vi "CheckTestSelection.vi"(3 "错误输入":errorcluster, 4 "产品型号":refnum<vi>, 5 "测试结果":refnum<vi>[](array[refnum]), 6 "测试选择":refnum<vi>[](array[refnum])) -> (0 "错误输出":errorcluster, 1 "TestPara":cluster{"TestStep":string[], "Enable":bool[]}[](array[cluster]), 2 "ExcelNames":string[](array[string]))   [LabVIEW 2013]
uses:
  <vilib>/Utility/NIReport.llb/NI_report.lvclass
  <vilib>/Utility/NIReport.llb/Excel/NI_Excel.lvclass
panel:
  out "进度条":u8(slide) scale=0.0..100.0
  out "字符串":string="正在检查测试用例配置文件"
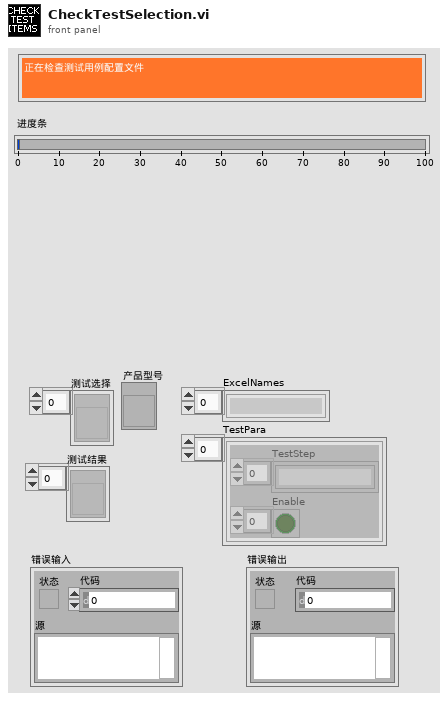
[diagram p1: front panel]
types:
  T1 = enum8{"Enabled", "Disabled", "Disabled and Grayed Out"}
  T2 = enum32{"invalid app kind", "Development System", "Run Time System", "Student Edition", "Embedded LabVIEW", "Evaluation", "Custom"}
  T3 = enum16{"maximized", "minimized", "normal", "no change"}
  T4 = enum16{"Standard Report", "HTML", "Word", "Excel"}
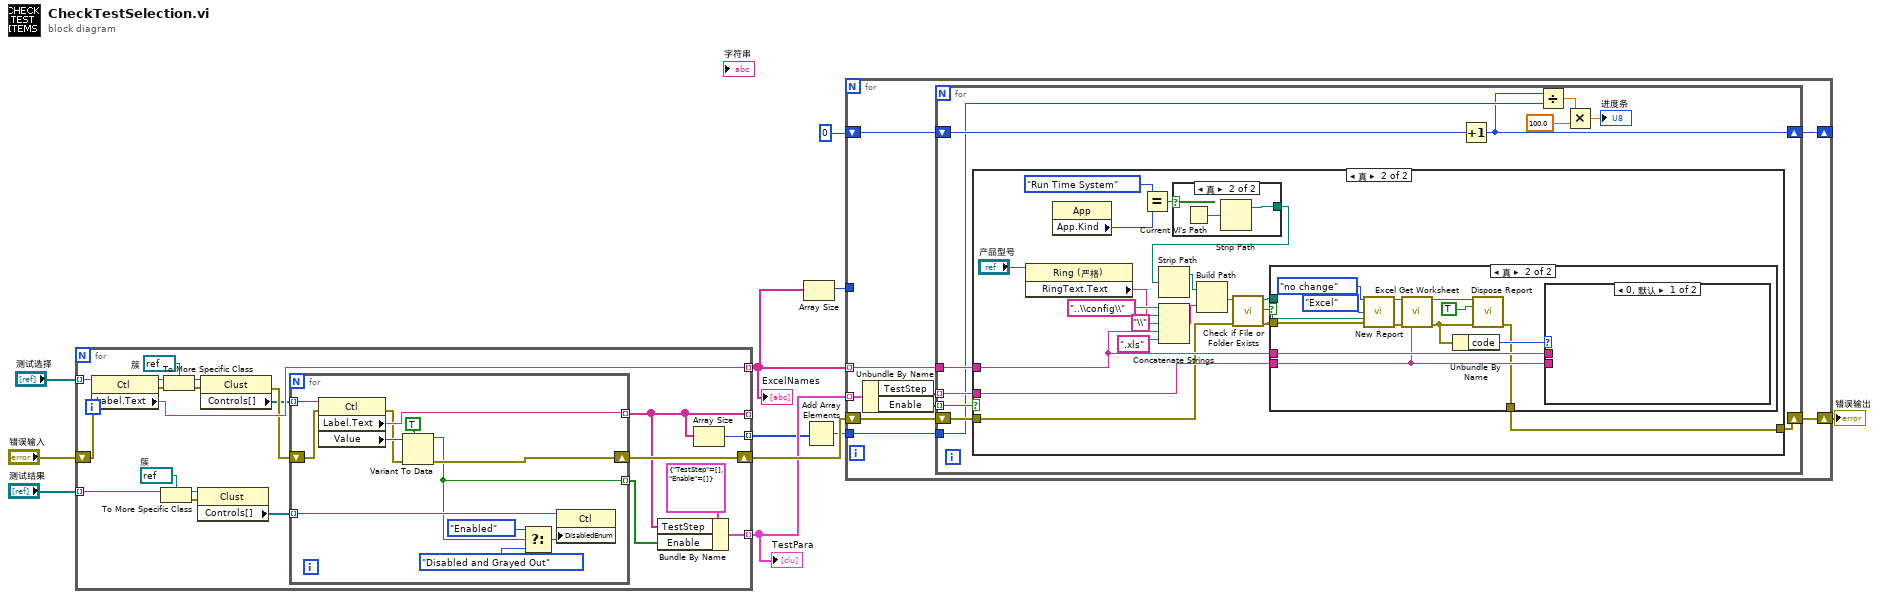
[diagram p0: block diagram]
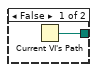
[diagram p3: hidden frame]
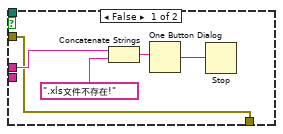
[diagram p4: hidden frame]
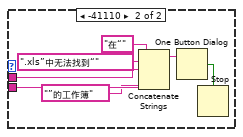
[diagram p5: hidden frame]
diagram:
  n1 = for {
    tunnel: "测试选择" -> [w32] mode=indexing
    tunnel: [w28] -> w5 mode=indexing
    tunnel: [w13] -> _ mode=indexing
    shift-right: [w23] -> w10
    shift-left: "错误输入" -> [w24]
    tunnel: "测试结果" -> [w19] mode=indexing
    tunnel: [w14] -> w6 mode=indexing
    tunnel: [w12] -> w2 mode=indexing
    w20 = refnum<vi> refnum  # 簇
    w30 = refnum<vi> refnum  # 簇
    n2 = property class="Ctl"(reference=w32, error in=w24) -> (reference out=w31:refnum<vi>, error out=w27:errorcluster, "Label.Text"=w28:string)
    n3 = To More Specific Class(target class=w20, reference=w19) -> (specific class reference=w21:refnum<vi>, error out=w22:errorcluster)  [unwired: 1 in]
    n4 = To More Specific Class(target class=w30, reference=w31, error in=w27) -> (specific class reference=w29:refnum<vi>, error out=w26:errorcluster)
    n5 = property class="Clust"(reference=w21, error in=w22) -> ("Controls[]"=w17:refnum<vi>[])  [unwired: 2 out]
    n6 = property class="Clust"(reference=w29, error in=w26) -> (error out=w25:errorcluster, "Controls[]"=w18:refnum<vi>[])  [unwired: 1 out]
    n7 = for {
      tunnel: w18 -> [w44] mode=indexing
      tunnel: [w41] -> w13 mode=indexing
      shift-right: [w38] -> w23
      shift-left: w25 -> [w40]
      tunnel: w17 -> [w37] mode=indexing
      tunnel: [w34] -> w16 mode=indexing
      n8 = property class="Ctl"(reference=w44, error in=w40) -> (error out=w39:errorcluster, "Label.Text"=w41:string, "Value"=w42:variant)  [unwired: 1 out]
      n9 = Variant To Data(error in=w39, type=TRUE, Variant=w42) -> (data=w34:bool, error out=w38:errorcluster)
      n10 = Select(t=T1."Enabled" ("禁用"), s=w34, f=T1."Disabled and Grayed Out" ("禁用")) -> (s? t:f=w33:T1)
      n11 = property class="Ctl"(reference=w37, "DisabledEnum"=w33) -> ()  [unwired: 1 in, 2 out]
    }
    n12 = Bundle By Name(cluster=cluster{"TestStep":string[], "Enable":bool[]} {"TestStep"=[], "Enable"=[]} ("簇"), "TestStep"=w13, "Enable"=w16) -> (w14:cluster{"TestStep":string[], "Enable":bool[]})
    n13 = Array Size(array=w13) -> (size(s)=w12:i32)
  }
  "ExcelNames" <- w5
  "TestPara" <- w6
  n14 = Array Size(array=w5) -> (size(s)=w4:i32)
  n15 = Add Array Elements(numeric array=w2) -> (sum=w1:i32)
  n16 = for {
    tunnel: w5 -> [w53] mode=indexing
    shift-right: [w51] -> w9
    shift-left: w10 -> [w52]
    tunnel: w6 -> [w50] mode=indexing
    tunnel: w4 -> [_]
    shift-right: [w46] -> _
    shift-left: 0 -> [w47]
    tunnel: w1 -> [w45]
    n17 = Unbundle By Name(w50) -> ("TestStep"=w49:string[], "Enable"=w48:bool[])
    n18 = for {
      tunnel: w53 -> [w64]
      shift-right: [w62] -> w51
      shift-left: w52 -> [w63]
      tunnel: w49 -> [w61] mode=indexing
      tunnel: w48 -> [w60] mode=indexing
      shift-right: [w54] -> w46
      shift-left: w47 -> [w59]
      tunnel: w45 -> [w55]
      n19 = case shown="真" w60 {
        tunnel: w64 -> [_ w76]
        tunnel: w61 -> [_ w75]
        tunnel: w63 -> [w65 w74]
        tunnel: [w65 w73] -> w62
        frame False {
        }
        frame True {
          n20 = property class="Ring (严格)"(reference="产品型号") -> ("RingText.Text"=w68:string)  [unwired: 1 in, 2 out]
          n21 = property class="App"() -> ("App.Kind"=w71:T2)  [unwired: 2 in, 2 out]
          n22 = Equal?(x=T2."Run Time System" ("y"), y=w71) -> (x = y?=w70:bool)
          n23 = Concatenate Strings("..\\config\\" ("连接的字符串"), w68, "\\" ("字符串"), w76, ".xls" ("连接的字符串")) -> (w79:string)
          n24 = case shown="真" w70 {
            tunnel: [w85 w87] -> w69
            frame False {
              n25 = Current VI's Path() -> (path=w85:path)
            }
            frame True {
              n26 = Current VI's Path() -> (path=w86:path)
              n27 = Strip Path(path=w86) -> (stripped path=w87:path)  [unwired: 1 out]
            }
          }
          n28 = Strip Path(path=w69) -> (stripped path=w81:path)  [unwired: 1 out]
          n29 = Build Path(base path=w81, name or relative path=w79) -> (appended path=w78:path)
          n30 = call <vilib>:"Check if File or Folder Exists.vi"("error in (no error)"=w74, "path"=w78) -> ("error out"=w84:errorcluster, "file or folder exists?"=w83:bool, "dup path"=w82:path)  [unwired: 7 out]
          n31 = case shown="真" w83 {
            tunnel: w84 -> [w88 w99]
            tunnel: w82 -> [_ w100]
            tunnel: w76 -> [w90 w98]
            tunnel: w75 -> [_ w97]
            tunnel: [w88 w93] -> w73
            frame False {
              n32 = Concatenate Strings(w90, ".xls文件不存在!" ("消息")) -> (w91:string)
              n33 = One Button Dialog(message=w91) -> (true=w89:bool)  [unwired: 1 in]
              n34 = Stop(stop? (T)=w89) -> ()
            }
            frame True {
              n35 = call <vilib>:"New Report.vi"("window state (normal)"=T3."no change", "report type"=T4."Excel", "template (empty)"=w100, "error in (no error)"=w99) -> ("report out"=w103:refnum<class "NI_report.lvclass">, "error out"=w102:errorcluster)  [unwired: 2 in, 8 out]
              n36 = call <vilib>:"Excel Get Worksheet.vi"("report in"=w103, "error in (no error)"=w102, "name (\"\")"=w97) -> ("report out"=w95:refnum<class "NI_report.lvclass">, "error out"=w96:errorcluster)  [unwired: 11 in]
              n37 = Unbundle By Name(w96) -> ("code"=w101:i32)
              n38 = call-dynamic "Dispose Report.vi"("report in"=w95, "wait until printing completed? (T)"=TRUE, "error in (no error)"=w96) -> ("error out"=w93:errorcluster)  [unwired: 2 in, 10 out]
              n39 = case shown="0, 默认" w101 {
                tunnel: w98 -> [_ w111]
                tunnel: w97 -> [_ w109]
                frame 0, Default {
                }
                frame -41110 {
                  n40 = Concatenate Strings("在“" ("连接的字符串"), w111, ".xls”中无法找到“" ("字符串"), w109, "”的工作簿" ("字符串")) -> (w107:string)
                  n41 = One Button Dialog(message=w107) -> (true=w106:bool)  [unwired: 1 in]
                  n42 = Stop(stop? (T)=w106) -> ()
                }
              }
            }
          }
        }
      }
      n43 = Increment(x=w59) -> (x+1=w54:i32)
      n44 = Divide(x=w54, y=w55) -> (x/y=w56:dbl)
      n45 = Multiply(x=w56, y=100.0) -> (x*y=→"进度条":dbl)
    }
  }
  "错误输出" <- w9
